vi "Pack Mutexed Publish Request.vi"(6 "Return Error Transport":refnum<class "ITransport.lvclass">, 7 "Publisher ID":string, 8 "PublicationPolicy":refnum<class "IPublicationPolicy.lvclass">, 9 "Publish Time (Use Current Time)":timestamp, 10 "Datum Value or Type":variant, 11 "Datum Name":string) -> (3 "MutexedPublishRequest Out":refnum<class "MutexedPublishRequest.lvclass">)   [LabVIEW 2017, in "IMediator.lvlib" / "MutexedPublishRequest.lvclass"]
uses:
  MutexedPublishRequest.lvclass
  C:/Git/mva-framework/Framework/IMediator/PublishRequest/PublishRequest.lvclass
  IPublicationPolicy/IPublicationPolicy.lvclass
  ITransport/ITransport.lvclass
  PublishRequest/PublishRequest.lvclass/PublishRequest.ctl
  MutexedPublishRequest.lvclass/MutexedPublishRequest.ctl
  PublishRequest/PublishRequest.lvclass
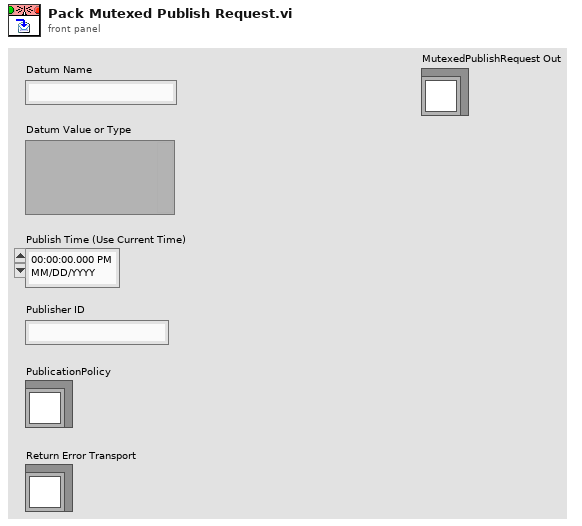
[diagram p1: front panel]
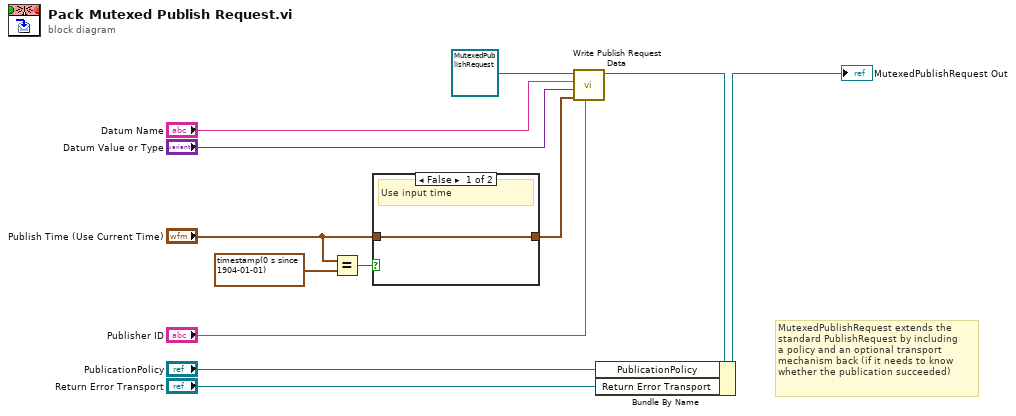
[diagram p0: block diagram]
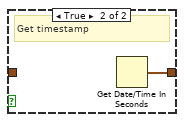
[diagram p2: hidden frame]
diagram:
  # "MutexedPublishRequest extends the\nstandard PublishRequest by including\na policy and an optional transport\nmechanism back (if it needs to know\nwhether the publication succeeded)"
  n1 = Equal?(x="Publish Time (Use Current Time)", y=timestamp(0 s since 1904-01-01)) -> (x = y?=w11:bool)
  n2 = case shown="False" w11 {
    tunnel: "Publish Time (Use Current Time)" -> [w13 _]
    tunnel: [w13 w14] -> w6
    frame False {
      # "Use input time"
    }
    frame True {
      # "Get timestamp"
      n3 = Get Date/Time In Seconds() -> (seconds since 1Jan1904=w14:timestamp)
    }
  }
  n4 = call "Write Publish Request Data.vi"("Publisher ID"="Publisher ID", "Publication Time"=w6, "Value"="Datum Value or Type", "Datum Name"="Datum Name", "PublishRequest In"=refnum<class "MutexedPublishRequest.lvclass"> refnum ("PublishRequest in")) -> ("PublishRequest Out"=w4:refnum<class "MutexedPublishRequest.lvclass">)  [unwired: 6 in]
  n5 = Bundle By Name(cluster=w4, "PublicationPolicy"="PublicationPolicy", "Return Error Transport"="Return Error Transport") -> (→"MutexedPublishRequest Out":refnum<class "MutexedPublishRequest.lvclass">)
